vi "Begin.vi"() -> (0 "error out":errorcluster)   [LabVIEW 2020]
doc: "Called before other user functions, this VI is expected to open initial I/O refnums, load in file data, and do all program initialization. Notice that the <B>error out</B> terminal is simply used for data flow. Wiring it to other structures or subVIs ensures that this VI runs first."
uses:
  <vilib>/Rock Robotics/WPI/DriverStation/WPI_DriverStationRobotMode2.ctl
  <vilib>/Rock Robotics/WPI/ThirdParty/Phoenix-LabVIEW/Motor Controller/Controls/CTRE_Phoenix_MotorControl_NeutralMode.ctl
  Robot Global Data.vi
panel:
  in  "error in":errorcluster
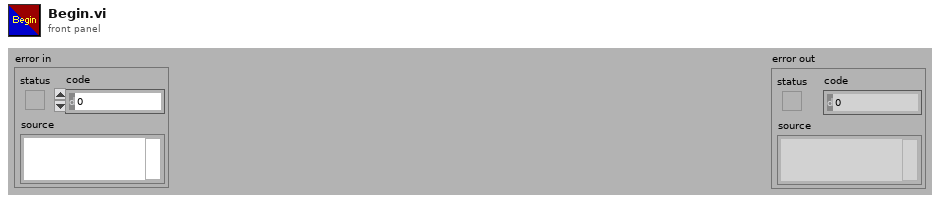
[diagram p1: front panel]
types:
  T1 = typedef "CTRE_Phoenix_MotorControl_NeutralMode.ctl" = enum8{"EEPROMSetting", "Override to Coast", "Override to Brake"}
  T2 = typedef "WPI_DriverStationRobotMode2.ctl" = enum16{"Autonomous Disabled", "Autonomous Enabled", "Teleop Disabled", "Teleop Enabled", "Disconnected", "Finish", "Test Disabled", "Test Enabled", "Emergency Stopped"}
  T3 = typedef "WPI_MotorControlDeviceRef.ctl" = cluster{"DeviceStatus":errorcluster, "Type":T4, "PWM":cluster{"PWM Channel":T5, "DeadBand":T6}, "CAN":cluster{"Device Number":u8, "SetOutput VI Ref":variant, "GetOutput VI Ref":variant, "Enable VI Ref":variant, "Disable VI Ref":variant, "Data":variant}, "Invert":bool, "DIO PWM":cluster{"PWM \"Enable\" Channel":T5, "DIOChannel":T7, "PWM Rate":dbl}}
  T4 = typedef "WPI_MotorControlType.ctl" = enum16{"PWM", "CAN", "DIO PWM"}
  T5 = typedef "FPGA_DIOPWMChannel.ctl" = enum8{"PWM 0", "PWM 1", "PWM 2", "PWM 3", "PWM 4", "PWM 5", "PWM 6", "PWM 7", "PWM 8", "PWM 9", "PWM MXP 0", "PWM MXP 1", "PWM MXP 2", "PWM MXP 3", "PWM MXP 4", "PWM MXP 5", "PWM MXP 6", "PWM MXP 7", "PWM MXP 8", "PWM MXP 9", "Invalid"}
  T6 = typedef "WPI_PWMDeadband.ctl" = cluster{"Name":string, "maxPositivePwm":i32, "minPositivePwm":i32, "centerPwm":i32, "maxNegativePwm":i32, "minNegativePwm":i32, "angularRange":u16}
  T7 = typedef "FPGA_DIOChannel.ctl" = enum8{"DIO 0", "DIO 1", "DIO 2", "DIO 3", "DIO 4", "DIO 5", "DIO 6", "DIO 7", "DIO 8", "DIO 9", "DIO MXP 0", "DIO MXP 1", "DIO MXP 2", "DIO MXP 3", "DIO MXP 4", "DIO MXP 5", "DIO MXP 6", "DIO MXP 7", "DIO MXP 8", "DIO MXP 9", "DIO MXP 10", "DIO MXP 11", "DIO MXP 12", "DIO MXP 13", "DIO MXP 14", "DIO MXP 15", "SPI Port CS1", "SPI Port CS2", "SPI Port CS3", "SPI Port MISO", "SPI Port MOSI", "Invalid"}
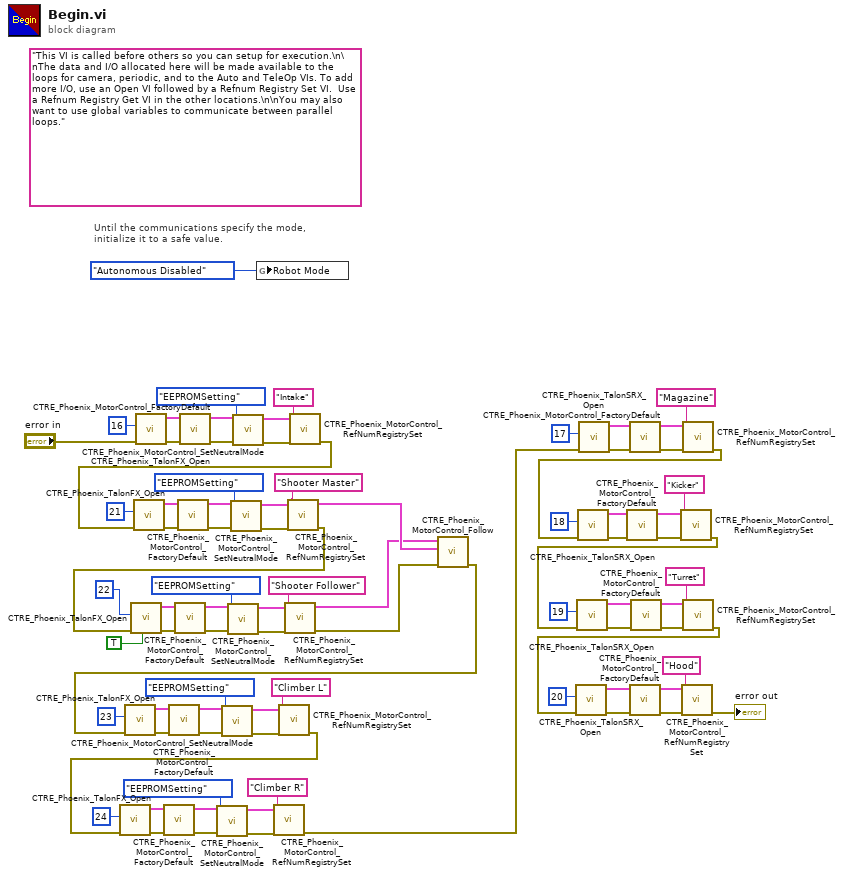
[diagram p0: block diagram]
diagram:
  (unwired) "This VI is called before others so you can setup for execution.\n\nThe data and I/O allocated here will be made available to the loops for camera, periodic, and to the Auto and TeleOp VIs. To add more I/O, use an Open VI followed by a Refnum Registry Set VI.  Use a Refnum Registry Get VI in the other locations.\n\nYou may also want to use global variables to communicate between parallel loops."
  # "Until the communications specify the mode,\ninitialize it to a safe value."
  n1 = call <vilib>:"CTRE_Phoenix_TalonFX_Open.vi"("error in"="error in", "Device Number"=u8 16) -> ("error out"=w83:errorcluster, "PhoenixMotorControlDevRef"=w82:T3)  [unwired: 8 in]
  n2 = call <vilib>:"CTRE_Phoenix_MotorControl_FactoryDefault.vi"("error in"=w83, "PhoenixMotorControlDevRef"=w82) -> ("error out"=w78:errorcluster, "PhoenixMotorControlDevRef"=w79:T3)  [unwired: 8 in]
  n3 = call <vilib>:"CTRE_Phoenix_MotorControl_SetNeutralMode.vi"("error in (no error)"=w78, "Motor Control Neutral Mode"=CTRE_Phoenix_MotorControl_NeutralMode."EEPROMSetting", "PhoenixMotorControlDevRef"=w79) -> ("error out"=w76:errorcluster, "PhoenixMotorControlDevRef"=w77:T3)  [unwired: 7 in]
  n4 = global write "Robot Global Data.vi" "Robot Mode"(WPI_DriverStationRobotMode2."Autonomous Disabled" ("Robot Mode")) -> ()
  n5 = call <vilib>:"CTRE_Phoenix_MotorControl_RefNumRegistrySet.vi"("error in (no error)"=w76, "refnum name"="Intake", "PhoenixMotorControlDevRef"=w77) -> ("error out"=w64:errorcluster)  [unwired: 7 in, 1 out]
  n6 = call <vilib>:"CTRE_Phoenix_TalonFX_Open.vi"("error in"=w64, "Device Number"=u8 21) -> ("error out"=w73:errorcluster, "PhoenixMotorControlDevRef"=w72:T3)  [unwired: 8 in]
  n7 = call <vilib>:"CTRE_Phoenix_MotorControl_FactoryDefault.vi"("error in"=w73, "PhoenixMotorControlDevRef"=w72) -> ("error out"=w68:errorcluster, "PhoenixMotorControlDevRef"=w69:T3)  [unwired: 8 in]
  n8 = call <vilib>:"CTRE_Phoenix_MotorControl_SetNeutralMode.vi"("error in (no error)"=w68, "Motor Control Neutral Mode"=CTRE_Phoenix_MotorControl_NeutralMode."EEPROMSetting", "PhoenixMotorControlDevRef"=w69) -> ("error out"=w66:errorcluster, "PhoenixMotorControlDevRef"=w67:T3)  [unwired: 7 in]
  n9 = call <vilib>:"CTRE_Phoenix_MotorControl_RefNumRegistrySet.vi"("error in (no error)"=w66, "refnum name"="Shooter Master", "PhoenixMotorControlDevRef"=w67) -> ("error out"=w54:errorcluster, "PhoenixMotorControlDevRef"=w53:T3)  [unwired: 7 in]
  n10 = call <vilib>:"CTRE_Phoenix_TalonFX_Open.vi"("Invert"=TRUE, "error in"=w54, "Device Number"=u8 22) -> ("error out"=w63:errorcluster, "PhoenixMotorControlDevRef"=w62:T3)  [unwired: 7 in]
  n11 = call <vilib>:"CTRE_Phoenix_MotorControl_FactoryDefault.vi"("error in"=w63, "PhoenixMotorControlDevRef"=w62) -> ("error out"=w58:errorcluster, "PhoenixMotorControlDevRef"=w59:T3)  [unwired: 8 in]
  n12 = call <vilib>:"CTRE_Phoenix_MotorControl_SetNeutralMode.vi"("error in (no error)"=w58, "Motor Control Neutral Mode"=CTRE_Phoenix_MotorControl_NeutralMode."EEPROMSetting", "PhoenixMotorControlDevRef"=w59) -> ("error out"=w56:errorcluster, "PhoenixMotorControlDevRef"=w57:T3)  [unwired: 7 in]
  n13 = call <vilib>:"CTRE_Phoenix_MotorControl_RefNumRegistrySet.vi"("error in (no error)"=w56, "refnum name"="Shooter Follower", "PhoenixMotorControlDevRef"=w57) -> ("error out"=w51:errorcluster, "PhoenixMotorControlDevRef"=w52:T3)  [unwired: 7 in]
  n14 = call <vilib>:"CTRE_Phoenix_MotorControl_Follow.vi"("error in (no error)"=w51, "Master Controller to Follow"=w53, "PhoenixMotorControlDevRef"=w52) -> ("error out"=w41:errorcluster)  [unwired: 7 in, 1 out]
  n15 = call <vilib>:"CTRE_Phoenix_TalonFX_Open.vi"("error in"=w41, "Device Number"=u8 23) -> ("error out"=w50:errorcluster, "PhoenixMotorControlDevRef"=w49:T3)  [unwired: 8 in]
  n16 = call <vilib>:"CTRE_Phoenix_MotorControl_FactoryDefault.vi"("error in"=w50, "PhoenixMotorControlDevRef"=w49) -> ("error out"=w45:errorcluster, "PhoenixMotorControlDevRef"=w46:T3)  [unwired: 8 in]
  n17 = call <vilib>:"CTRE_Phoenix_MotorControl_SetNeutralMode.vi"("error in (no error)"=w45, "Motor Control Neutral Mode"=CTRE_Phoenix_MotorControl_NeutralMode."EEPROMSetting", "PhoenixMotorControlDevRef"=w46) -> ("error out"=w43:errorcluster, "PhoenixMotorControlDevRef"=w44:T3)  [unwired: 7 in]
  n18 = call <vilib>:"CTRE_Phoenix_MotorControl_RefNumRegistrySet.vi"("error in (no error)"=w43, "refnum name"="Climber L", "PhoenixMotorControlDevRef"=w44) -> ("error out"=w31:errorcluster)  [unwired: 7 in, 1 out]
  n19 = call <vilib>:"CTRE_Phoenix_TalonFX_Open.vi"("error in"=w31, "Device Number"=u8 24) -> ("error out"=w40:errorcluster, "PhoenixMotorControlDevRef"=w39:T3)  [unwired: 8 in]
  n20 = call <vilib>:"CTRE_Phoenix_MotorControl_FactoryDefault.vi"("error in"=w40, "PhoenixMotorControlDevRef"=w39) -> ("error out"=w35:errorcluster, "PhoenixMotorControlDevRef"=w36:T3)  [unwired: 8 in]
  n21 = call <vilib>:"CTRE_Phoenix_MotorControl_SetNeutralMode.vi"("error in (no error)"=w35, "Motor Control Neutral Mode"=CTRE_Phoenix_MotorControl_NeutralMode."EEPROMSetting", "PhoenixMotorControlDevRef"=w36) -> ("error out"=w33:errorcluster, "PhoenixMotorControlDevRef"=w34:T3)  [unwired: 7 in]
  n22 = call <vilib>:"CTRE_Phoenix_MotorControl_RefNumRegistrySet.vi"("error in (no error)"=w33, "refnum name"="Climber R", "PhoenixMotorControlDevRef"=w34) -> ("error out"=w29:errorcluster)  [unwired: 7 in, 1 out]
  n23 = call <vilib>:"CTRE_Phoenix_TalonSRX_Open.vi"("error in"=w29, "Device Number"=u8 17) -> ("error out"=w28:errorcluster, "PhoenixMotorControlDevRef"=w27:T3)  [unwired: 8 in]
  n24 = call <vilib>:"CTRE_Phoenix_MotorControl_FactoryDefault.vi"("error in"=w28, "PhoenixMotorControlDevRef"=w27) -> ("error out"=w20:errorcluster, "PhoenixMotorControlDevRef"=w19:T3)  [unwired: 8 in]
  n25 = call <vilib>:"CTRE_Phoenix_MotorControl_RefNumRegistrySet.vi"("error in (no error)"=w20, "refnum name"="Magazine", "PhoenixMotorControlDevRef"=w19) -> ("error out"=w4:errorcluster)  [unwired: 7 in, 1 out]
  n26 = call <vilib>:"CTRE_Phoenix_TalonSRX_Open.vi"("error in"=w4, "Device Number"=u8 18) -> ("error out"=w26:errorcluster, "PhoenixMotorControlDevRef"=w25:T3)  [unwired: 8 in]
  n27 = call <vilib>:"CTRE_Phoenix_MotorControl_FactoryDefault.vi"("error in"=w26, "PhoenixMotorControlDevRef"=w25) -> ("error out"=w18:errorcluster, "PhoenixMotorControlDevRef"=w17:T3)  [unwired: 8 in]
  n28 = call <vilib>:"CTRE_Phoenix_MotorControl_RefNumRegistrySet.vi"("error in (no error)"=w18, "refnum name"="Kicker", "PhoenixMotorControlDevRef"=w17) -> ("error out"=w3:errorcluster)  [unwired: 7 in, 1 out]
  n29 = call <vilib>:"CTRE_Phoenix_TalonSRX_Open.vi"("error in"=w3, "Device Number"=u8 19) -> ("error out"=w24:errorcluster, "PhoenixMotorControlDevRef"=w23:T3)  [unwired: 8 in]
  n30 = call <vilib>:"CTRE_Phoenix_MotorControl_FactoryDefault.vi"("error in"=w24, "PhoenixMotorControlDevRef"=w23) -> ("error out"=w16:errorcluster, "PhoenixMotorControlDevRef"=w15:T3)  [unwired: 8 in]
  n31 = call <vilib>:"CTRE_Phoenix_MotorControl_RefNumRegistrySet.vi"("error in (no error)"=w16, "refnum name"="Turret", "PhoenixMotorControlDevRef"=w15) -> ("error out"=w2:errorcluster)  [unwired: 7 in, 1 out]
  n32 = call <vilib>:"CTRE_Phoenix_TalonSRX_Open.vi"("error in"=w2, "Device Number"=u8 20) -> ("error out"=w22:errorcluster, "PhoenixMotorControlDevRef"=w21:T3)  [unwired: 8 in]
  n33 = call <vilib>:"CTRE_Phoenix_MotorControl_FactoryDefault.vi"("error in"=w22, "PhoenixMotorControlDevRef"=w21) -> ("error out"=w14:errorcluster, "PhoenixMotorControlDevRef"=w13:T3)  [unwired: 8 in]
  n34 = call <vilib>:"CTRE_Phoenix_MotorControl_RefNumRegistrySet.vi"("error in (no error)"=w14, "refnum name"="Hood", "PhoenixMotorControlDevRef"=w13) -> ("error out"=→"error out":errorcluster)  [unwired: 7 in, 1 out]
